vi "test_U32 Write and Read.vi"(8 "error in (no error)":errorcluster, 11 "Scalar Channels Testing in":refnum<class "FPGA Addon Scalar Channels System Tests.lvclass">) -> (0 "error out":errorcluster, 3 "Scalar Channels Testing out":refnum<class "FPGA Addon Scalar Channels System Tests.lvclass">)   [LabVIEW 2018, in "FPGA Addon Scalar Channels System Tests.lvclass"]
uses:
  FPGA Addon Scalar Channels System Tests.lvclass
  D:/GitBranches/niveristand-fpga-addon-custom-device/Source/Tests/FPGA Addon Test Class/FPGA Addon Test Class.lvclass
  D:/GitBranches/niveristand-custom-device-testing-tools/VeriStandTestCase/VeriStandTestCase.lvclass
  FPGA Addon Test Class/FPGA Addon Test Class.lvclass/FPGA Addon Test Class.ctl
  FPGA Addon Test Class/FPGA Addon Test Class.lvclass
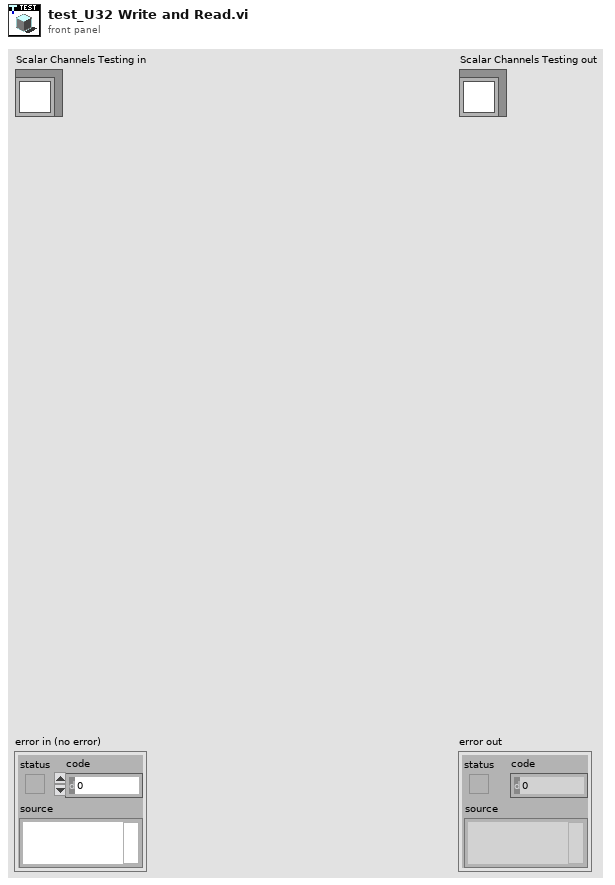
[diagram p1: front panel]
types:
  T1 = typedef "NI_VS Workspace ExecutionAPI.lvlib/WorkspaceAPI.ctl" = refnum<k24>
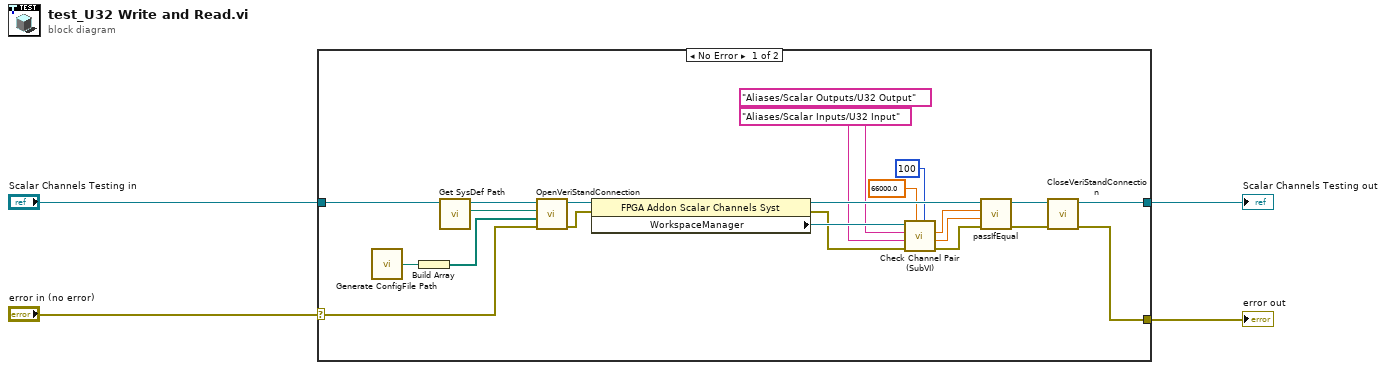
[diagram p0: block diagram]
diagram:
  n1 = case shown="No Error" "error in (no error)" {
    selector: "error in (no error)" -> [w19 w28]
    tunnel: [w25 w28] -> w3
    tunnel: [w26 w27] -> w1
    tunnel: "Scalar Channels Testing in" -> [w18 w27]
    frame No Error {
      n2 = call "Generate ConfigFile Path.vi"() -> ("ConfigFile path"=w6:path)
      n3 = Build Array(w6) -> (w5:path[])
      n4 = call "Get SysDef Path.vi"("Scalar Channels Testing in"=w18) -> ("SysDef Path"=w16:path, "Scalar Channels Testing out"=w17:refnum<class "FPGA Addon Scalar Channels System Tests.lvclass">)  [unwired: 9 in]
      n5 = call-dynamic "OpenVeriStandConnection.vi"("error in (no error)"=w19, "overrides files"=w5, "System Definition File"=w16, "VeriStand Test Case in"=w17) -> ("error out"=w24:errorcluster, "VeriStand Test Case out"=w23:refnum<class "FPGA Addon Scalar Channels System Tests.lvclass">)  [unwired: 5 in, 1 out]
      n6 = property class="FPGA Addon Scalar Channels Syst"(reference=w23, error in=w24) -> (reference out=w22:refnum<class "FPGA Addon Scalar Channels System Tests.lvclass">, error out=w11:errorcluster, "WorkspaceManager"=w15:T1)
      n7 = call "Check Channel Pair (SubVI).vi"("milliseconds to wait"=u32 100, "Test Value"=66000.0 ("Value"), "error in (no error)"=w11, "Input Channel"="Aliases/Scalar Inputs/U32 Input" ("Channel"), "Output Channel"="Aliases/Scalar Outputs/U32 Output" ("Channel"), "WorkspaceManager in"=w15) -> ("error out"=w12:errorcluster, "InputChannel Value"=w7:dbl, "OutputChannel Value"=w8:dbl)  [unwired: 2 in, 1 out]
      n8 = call-dynamic "passIfEqual.vi"("error in (no error)"=w12, "y"=w7, "x"=w8, "TestCase in"=w22) -> ("error out"=w20:errorcluster, "TestCase out"=w21:refnum<class "FPGA Addon Scalar Channels System Tests.lvclass">)  [unwired: 6 in]
      n9 = call-dynamic "CloseVeriStandConnection.vi"("error in (no error)"=w20, "VeriStand Test Case in"=w21) -> ("error out"=w25:errorcluster, "VeriStand Test Case out"=w26:refnum<class "FPGA Addon Scalar Channels System Tests.lvclass">)  [unwired: 8 in]
    }
    frame Error {
    }
  }
  "error out" <- w3
  "Scalar Channels Testing out" <- w1
